vi "PH_Beckhoff-16BB.handle PA Chiller.vi"(0 "i ref in":refnum<vi>, 2 "Current Digital Inputs":T1, 3 "changed DE Values":i32[](array[numeric]), 5 "error in":errorcluster) -> (14 "i ref out":refnum<vi>, 19 "error out":errorcluster)   [LabVIEW 2014, in "PH_Beckhoff-16BB.lvlib"]
doc: "This VI handles the incoming information about PA Chiller inputs: The status is calculated and, if it changed, set to own attributes and published via DIM. All information is indicated at the GUI."
uses:
  PH_Beckhoff-16BB.lvlib
  PH_Beckhoff/PH_Beckhoff.Digital Inputs.ctl
  PH_StatusHandler/PH_StatusHandler.Status.ctl
  PH_Common/PH_Common.lvlib
  PH_StatusHandler/PH_StatusHandler.lvlib
  PH_Beckhoff/PH_Beckhoff.lvlib
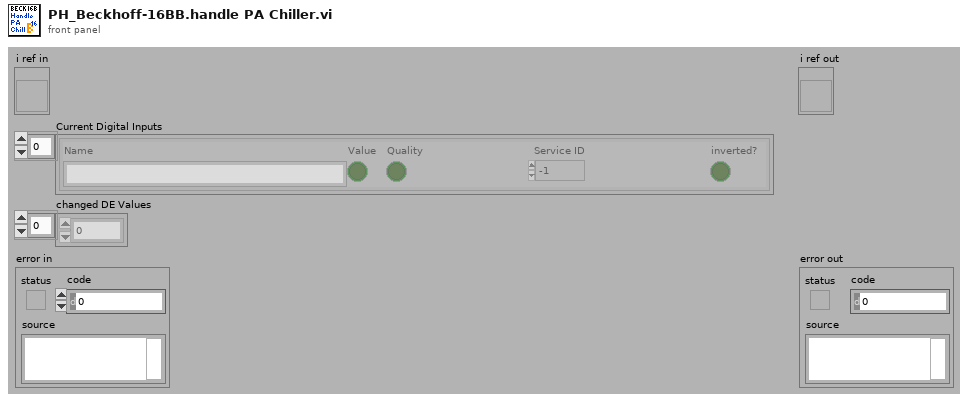
[diagram p1: front panel]
types:
  T1 = typedef "PH_Beckhoff.lvlib/PH_Beckhoff.Digital Inputs.ctl" = cluster{"Name":string, "Value":bool, "Quality":bool, "Service ID":i32, "inverted?":bool}[]
  T2 = typedef "PH_Beckhoff-16BB.lvlib/PH_Beckhoff-16BB.i attribute.ctl" = cluster{"PA Chiller":cluster{"PSDB":cluster{"Status Service ID":i32, "Instance ID":i32, "Data Status":T3, "Ref Status":refnum<vi>, "Error Code":i32}, "Status":cluster{"GUI Ref":refnum<vi>, "Status Service ID":i32, "Status":T4}, "DIs":cluster{"Flow Control":cluster{"GUI Ref":refnum<vi>, "# in Data":i32}, "High-Temp":cluster{"GUI Ref":refnum<vi>, "# in Data":i32}, "Conductivity":cluster{"GUI Ref":refnum<vi>, "# in Data":i32}, "Niveau":cluster{"GUI Ref":refnum<vi>, "# in Data":i32}}, "PSDB Thread":cluster{"Ref":refnum<vi>, "Q-Ref":refnum<queue>}}, "PSDB":cluster{"Shot #":i32, "Subsystem":T5}, "Racktype":string, "PSDB Credentials":T6}
  T3 = typedef "PH_PSDBWriter.lvlib/PH_PSDBWriter.Data Status.ctl" = i16
  T4 = typedef "PH_StatusHandler.lvlib/PH_StatusHandler.Status.ctl" = i16
  T5 = typedef "PH_PSDBWriter.lvlib/PH_PSDBWriter.PHELIX-Subsystems.ctl" = i32
  T6 = typedef "PH_Common.lvlib/PH_Connection.PSDB Credentials.ctl" = cluster{"PW":string, "ID":string, "DS":string}
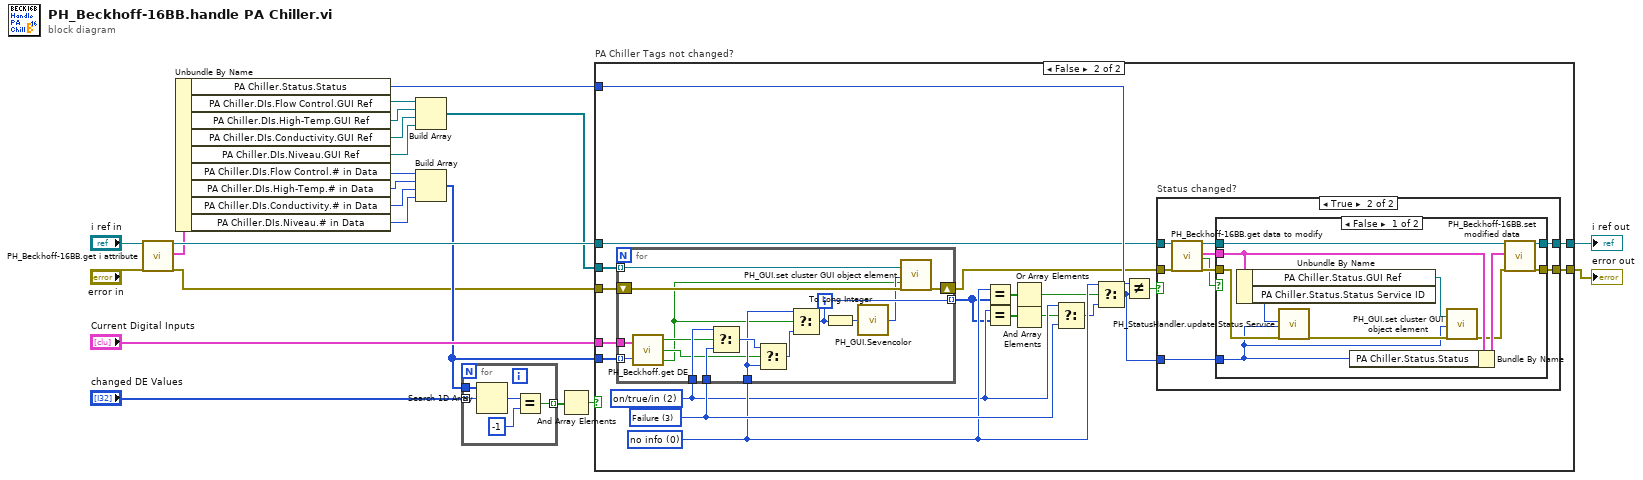
[diagram p0: block diagram]
diagram:
  n1 = call "PH_Beckhoff-16BB.get i attribute.vi"("i ref in"="i ref in", "error in (no error)"="error in") -> ("i ref out"=w19:refnum<vi>, "i attribute"=w17:T2, "error out"=w7:errorcluster)  [unwired: 15 in]
  n2 = Unbundle By Name(w17) -> ("PA Chiller.Status.Status"=w22:T4, "PA Chiller.DIs.Flow Control.GUI Ref"=w13:refnum<vi>, "PA Chiller.DIs.High-Temp.GUI Ref"=w12:refnum<vi>, "PA Chiller.DIs.Conductivity.GUI Ref"=w11:refnum<vi>, "PA Chiller.DIs.Niveau.GUI Ref"=w10:refnum<vi>, "PA Chiller.DIs.Flow Control.# in Data"=w4:i32, "PA Chiller.DIs.High-Temp.# in Data"=w3:i32, "PA Chiller.DIs.Conductivity.# in Data"=w2:i32, "PA Chiller.DIs.Niveau.# in Data"=w1:i32)
  n3 = Build Array(w13, w12, w11, w10) -> (w9:refnum<vi>[])
  n4 = Build Array(w4, w3, w2, w1) -> (w14:i32[])
  n5 = for {
    tunnel: w14 -> [w27]
    tunnel: "changed DE Values" -> [w26] mode=indexing
    tunnel: [w25] -> w6 mode=indexing
    n6 = Search 1D Array(1D array=w27, element=w26) -> (index of element=w24:i32)  [unwired: 1 in]
    n7 = Equal?(x=w24, y=-1) -> (x = y?=w25:bool)
  }
  n8 = And Array Elements(Boolean array=w6) -> (logical AND=w5:bool)
  n9 = case "PA Chiller Tags not changed?" shown="False" w5 {
    tunnel: w22 -> [_ w47]
    tunnel: w19 -> [w29 w37]
    tunnel: [w29 w36] -> w18
    tunnel: "Current Digital Inputs" -> [_ w35]
    tunnel: w14 -> [_ w34]
    tunnel: w9 -> [_ w33]
    tunnel: [w28 w32] -> w8
    tunnel: w7 -> [w28 w31]
    frame True {
    }
    frame False {
      w46 = T4 3 items=["no info", "off/false/out", "on/true/in", "Failure", "Alarm", "Status 1", "Status 2", "Status 3"] ("PA Chiller.Status")
      w44 = T4 2 items=["no info", "off/false/out", "on/true/in", "Failure", "Alarm", "Status 1", "Status 2", "Status 3"] ("PA Chiller.Status")
      w45 = T4 0 items=["no info", "off/false/out", "on/true/in", "Failure", "Alarm", "Status 1", "Status 2", "Status 3"] ("PA Chiller.Status")
      n10 = for {
        tunnel: [w84] -> w43 mode=indexing
        tunnel: w45 -> [w85]
        tunnel: w44 -> [w87]
        tunnel: w46 -> [w86]
        tunnel: w35 -> [w82]
        tunnel: w34 -> [w79] mode=indexing
        tunnel: w33 -> [w78] mode=indexing
        shift-right: [w77] -> w30
        shift-left: w31 -> [w76]
        n11 = call "PH_Beckhoff.get DE.vi"("Digital Values"=w82, "index of element"=w79) -> ("Value"=w81:bool, "Quality"=w80:bool, "Tag not found"=w74:bool)
        n12 = Select(t=w87, s=w81, f=w86) -> (s? t:f=w88:T4)
        n13 = Select(t=w88, s=w80, f=w85) -> (s? t:f=w89:T4)
        n14 = Select(t=w85, s=w74, f=w89) -> (s? t:f=w84:T4)
        n15 = To Long Integer(number=w84) -> (32bit integer=w83:i32)
        n16 = call "PH_GUI.Sevencolor.vi"("State"=w83) -> ("Color Box"=w75:u32)
        n17 = call "PH_GUI.set cluster GUI object element.vi"("Ctl Refnum"=w78, "Value"=w75, "Blinking? (false)"=w74, "error in"=w76) -> ("error out"=w77:errorcluster)  [unwired: 15 in]
      }
      n18 = Equal?(x=w45, y=w43) -> (x = y?=w38:bool[])
      n19 = Equal?(x=w44, y=w43) -> (x = y?=w40:bool[])
      n20 = Or Array Elements(Boolean array=w38) -> (logical OR=w39:bool)
      n21 = And Array Elements(Boolean array=w40) -> (logical AND=w41:bool)
      n22 = Select(t=w44, s=w41, f=w46) -> (s? t:f=w42:T4)
      n23 = Select(t=w45, s=w39, f=w42) -> (s? t:f=w49:T4)
      n24 = Not Equal?(x=w47, y=w49) -> (x != y?=w48:bool)
      n25 = case "Status changed?" shown="True" w48 {
        tunnel: w30 -> [w50 w60]
        tunnel: [w51 w59] -> w36
        tunnel: w37 -> [w51 w58]
        tunnel: [w50 w55] -> w32
        tunnel: w49 -> [_ w52]
        frame False {
        }
        frame True {
          n26 = call "PH_Beckhoff-16BB.get data to modify.vi"("i ref in"=w58, "error in (no error)"=w60) -> ("i ref out"=w57:refnum<vi>, "i attribute"=w53:T2, "timed out"=w54:bool, "error out"=w56:errorcluster)  [unwired: 14 in]
          n27 = case shown="False" w54 {
            tunnel: [w71 w73] -> w59
            tunnel: w57 -> [w70 w73]
            tunnel: w56 -> [w65 w72]
            tunnel: [w69 w72] -> w55
            tunnel: w53 -> [w67 _]
            tunnel: w52 -> [w62 _]
            frame False {
              n28 = Unbundle By Name(w67) -> ("PA Chiller.Status.GUI Ref"=w61:refnum<vi>, "PA Chiller.Status.Status Service ID"=w66:i32)
              n29 = call "PH_StatusHandler.update Status Service.vi"("Service ID"=w66, "Status"=w62, "error in (no error)"=w65) -> ("error out"=w64:errorcluster)  [unwired: 16 in]
              n30 = Bundle By Name(cluster=w67, "PA Chiller.Status.Status"=w62) -> (w68:T2)
              n31 = call "PH_GUI.set cluster GUI object element.vi"("Ctl Refnum"=w61, "Value"=w62, "error in"=w64) -> ("error out"=w63:errorcluster)  [unwired: 16 in]
              n32 = call "PH_Beckhoff-16BB.set modified data.vi"("i ref in"=w70, "i attribute"=w68, "error in (no error)"=w63) -> ("i ref out"=w71:refnum<vi>, "error out"=w69:errorcluster)  [unwired: 15 in]
            }
            frame True {
            }
          }
        }
      }
    }
  }
  "error out" <- w8
  "i ref out" <- w18
